vi "muParser Demo.vi"() -> ()   [LabVIEW 2015]
uses:
  muExpr/muExpr.lvclass/muExpr.ctl
  muExpr/Set Variable Value.vi
  muExpr/Eval.vi
  mupLib/mupSetVarValue.vi
  mupLib/mupEval.vi
  mupLib/mupCheckError.vi
  <vilib>/Utility/error.llb/Error Cluster From Error Code.vi
  muExpr/muExpr.lvclass
panel:
  in  "Constants":cluster{"name":string, "value":dbl}[](array[cluster])=[{"name"="a", "value"=1.0}, {"name"="b", "value"=2.0}]
  out "error out":errorcluster
  out "XY Graph":cluster{dbl[], dbl[]}(graph)
  in  "Iterations":i32=1000
  out "Variable Names":string[](array[string])
  in  "Variable (x)":string="x"
  in  "Expression":string="a*x+b"
  in  "varValues (initial)":dbl[](array[numeric])=[0.0, 0.0, 0.0, 0.0, 0.0, 0.0] format="%#_13g"
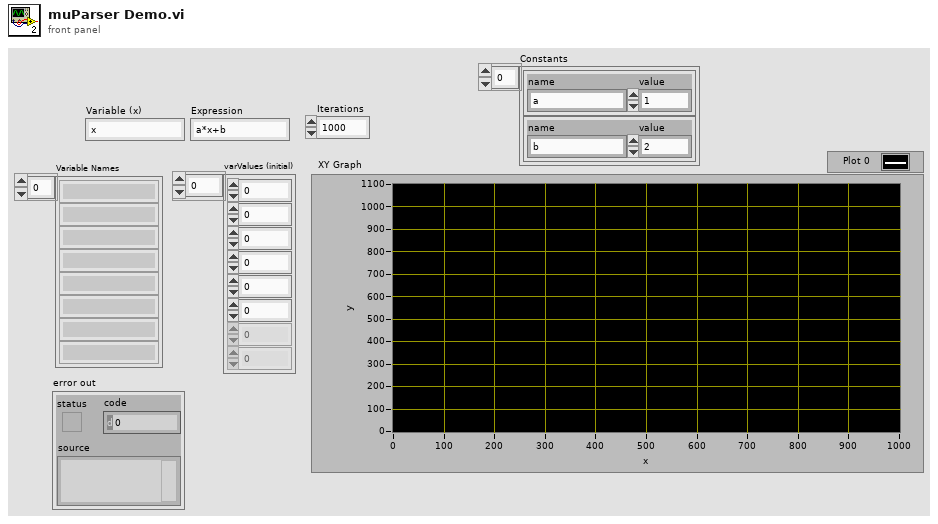
[diagram p1: front panel]
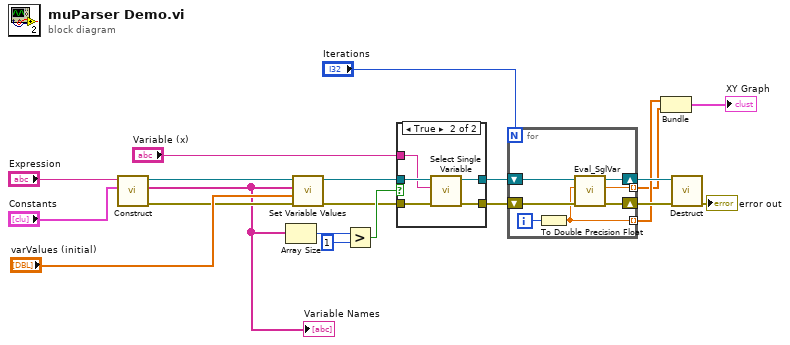
[diagram p0: block diagram]
diagram:
  n1 = call "Construct.vi"("Constants"="Constants", "Expression"="Expression") -> ("error out"=w19:errorcluster, "Variable Names"=w17:string[], "muExpr out"=w21:refnum<class "muExpr.lvclass">)  [unwired: 7 in]
  "Variable Names" <- w17
  n2 = Array Size(array=w17) -> (size(s)=w16:i32)
  n3 = call "Set Variable Values.vi"("error in (no error)"=w19, "varValues"="varValues (initial)", "varNames"=w17, "muExpr in"=w21) -> ("error out"=w12:errorcluster, "muExpr out"=w13:refnum<class "muExpr.lvclass">)  [unwired: 6 in]
  n4 = Greater?(x=w16, y=1) -> (0:w14:bool)
  n5 = case shown="True" w14 {
    tunnel: w13 -> [w23 w28]
    tunnel: w12 -> [w22 w27]
    tunnel: [w22 w26] -> w8
    tunnel: [w23 w25] -> w10
    tunnel: "Variable (x)" -> [_ w24]
    frame False {
    }
    frame True {
      n6 = call "Select Single Variable.vi"("error in (no error)"=w27, "varName"=w24, "muExpr in"=w28) -> ("error out"=w26:errorcluster, "muExpr out"=w25:refnum<class "muExpr.lvclass">)  [unwired: 7 in]
    }
  }
  n7 = for {
    N: "Iterations" -> [_]
    shift-right: [w34] -> w9
    shift-left: w10 -> [w35]
    shift-right: [w32] -> w7
    shift-left: w8 -> [w33]
    tunnel: [w30] -> w4 mode=indexing
    tunnel: [w29] -> w5 mode=indexing
    i -> [w31]
    n8 = To Double Precision Float(number=w31) -> (double precision float=w29:dbl)
    n9 = call "Eval_SglVar.vi"("error in (no error)"=w33, "varValue"=w29, "muExpr in"=w35) -> ("error out"=w32:errorcluster, "Result"=w30:dbl, "muExpr out"=w34:refnum<class "muExpr.lvclass">)  [unwired: 6 in]
  }
  n10 = Bundle(w5, w4) -> (→"XY Graph":cluster{dbl[], dbl[]})  [unwired: 1 in]
  n11 = call "Destruct.vi"("error in (no error)"=w7, "muExpr in"=w9) -> ("error out"=→"error out":errorcluster)  [unwired: 9 in]
